vi "Convert Distance to Encoder.vi"(5 "Dist (ft)":dbl) -> (2 "Encoder":dbl)   [LabVIEW 2014]
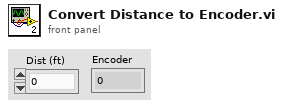
[diagram p1: front panel]
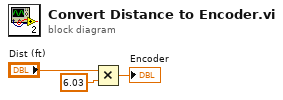
[diagram p0: block diagram]
diagram:
  n1 = Multiply(x="Dist (ft)", y=6.03) -> (x*y=→"Encoder":dbl)
